vi "SVPO RMS Level (1 Ch DBL WDT).vi"(6 "restart averaging? (F)":bool, 11 "scaled signal [EU]":waveform(dbl)={"t0"=timestamp(0 s since 1904-01-01), "dt"=0.0, "Y"=[]}) -> (3 "RMS level":dbl=nan, 4 "duration [s]":dbl, 5 "timestamp":timestamp)   [LabVIEW 2017, in "SoundVib_VibrationLevel.lvlib"]
doc: "Computes the root-mean-square (RMS) level of scaled time waveform signals and scaled array signals. <B>scaled signal [EU]</B> should have a zero DC component. You can attenuate the DC component with hardware AC-coupling filters and with software high-pass filters. Use this VI on embedded targets that have limited computational resources. Wire data to the <B>scaled signal [EU]</B> input to determine the polymorphic instance to use or manually select the instance."
uses:
  <vilib>/addons/Sound and Vibration/svt_Level/SoundVib_VibrationLevel.lvlib
  <vilib>/addons/Sound and Vibration/svt_Level/SVPO RMS Level (1 Ch DBL Array) with IC.vi
  <vilib>/Analysis/baseanly.llb/Dot Product.vi
  <vilib>/Analysis/baseanly.llb/Real Dot Product.vi
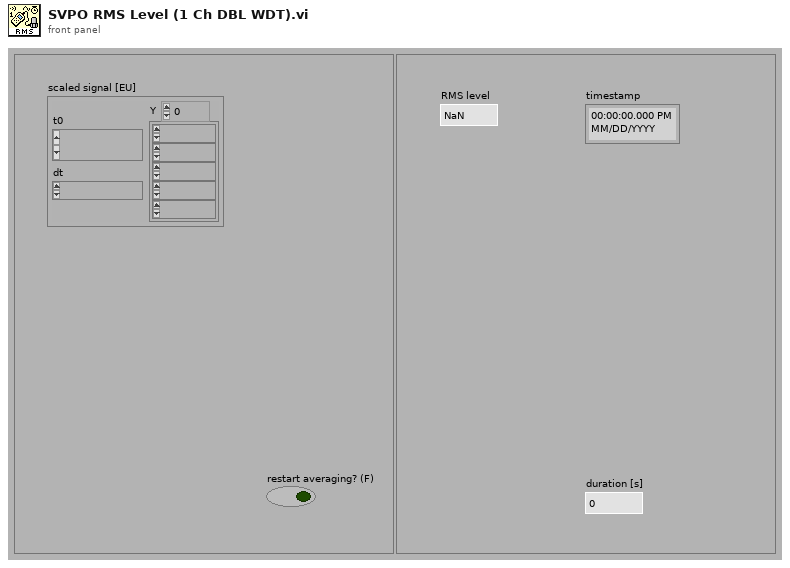
[diagram p1: front panel]
types:
  T1 = typedef "svc_RMS Level State.ctl" = cluster{"Squared Sum":dbl, "Size":u64, "timestamp":timestamp}
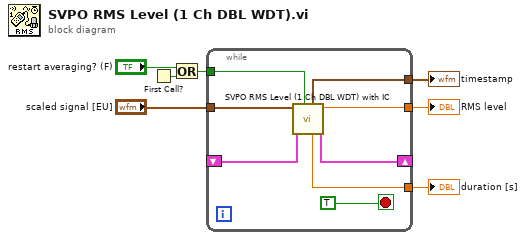
[diagram p0: block diagram]
diagram:
  n1 = First Call?() -> (First Call?: T/F=w6:bool)
  n2 = Or(x="restart averaging? (F)", y=w6) -> (x .or. y?=w4:bool)
  n3 = while {
    tunnel: w4 -> [w14]
    tunnel: "scaled signal [EU]" -> [w13]
    tunnel: [w10] -> w3
    tunnel: [w12] -> w2
    tunnel: [w11] -> w1
    shift-right: [w9] -> _
    shift-left: _ -> [w8]
    stop <- TRUE stop-if-true
    n4 = call <vilib>:"SVPO RMS Level (1 Ch DBL WDT) with IC.vi"("restart averaging? (F)"=w14, "initial conditions"=w8, "scaled signal [EU]"=w13) -> ("final conditions"=w9:T1, "RMS level"=w11:dbl, "duration [s]"=w10:dbl, "timestamp"=w12:timestamp)  [unwired: 5 in]
  }
  "RMS level" <- w1
  "timestamp" <- w2
  "duration [s]" <- w3
